vi "Subvi Notify User.vi"(1 "Imaging":bool, 2 "PresentCutsIn":u32, 3 "TotalCutsIn":u32, 4 "NotifyAbout":T1(ring)) -> (0 "Error":bool)   [LabVIEW 2012]
uses:
  ProSCI Global.vi
  <vilib>/Utility/SMTP/NI_SMTPEmail.lvlib
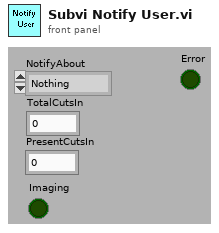
[diagram p1: front panel]
types:
  T1 = enum16{"Nothing", "In Progress", "Aborted", "Completed", "Sec TO"}
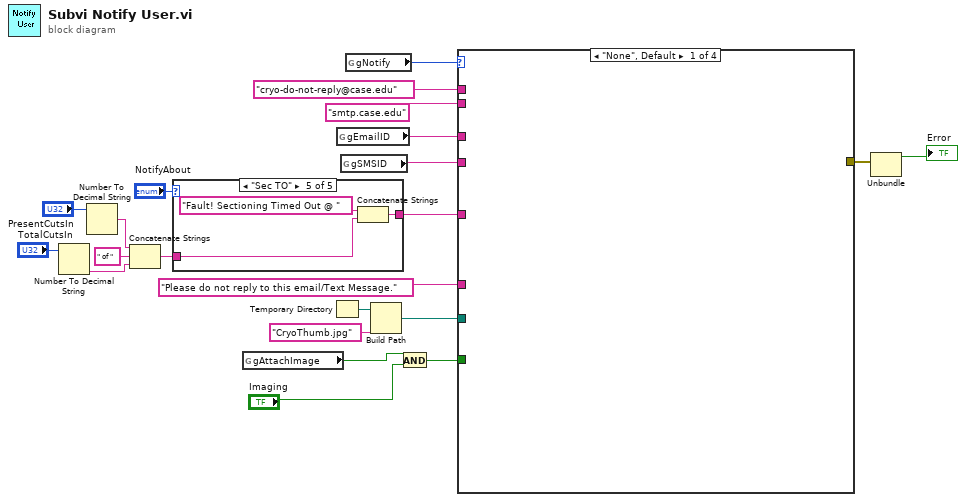
[diagram p0: block diagram]
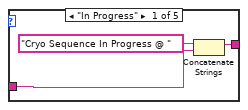
[diagram p2: hidden frame]
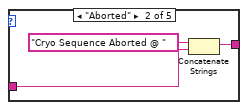
[diagram p3: hidden frame]
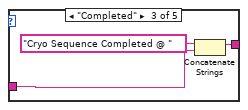
[diagram p4: hidden frame]
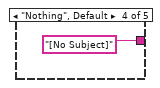
[diagram p5: hidden frame]
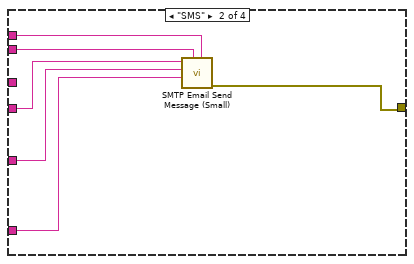
[diagram p6: hidden frame]
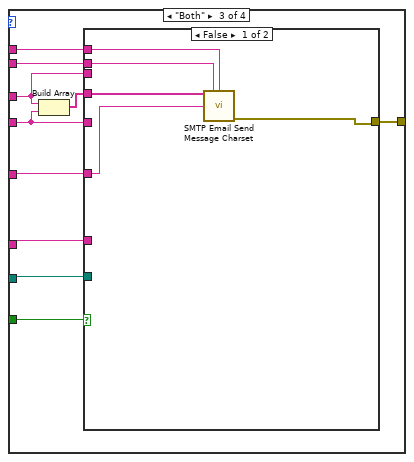
[diagram p7: hidden frame]
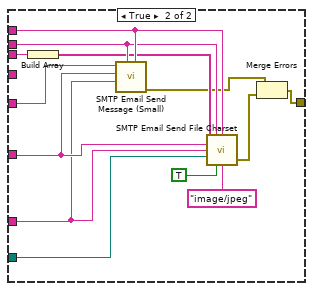
[diagram p8: hidden frame]
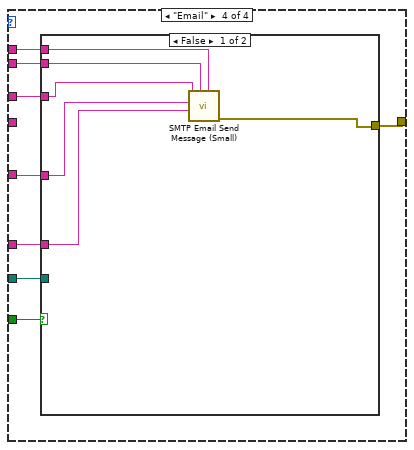
[diagram p9: hidden frame]
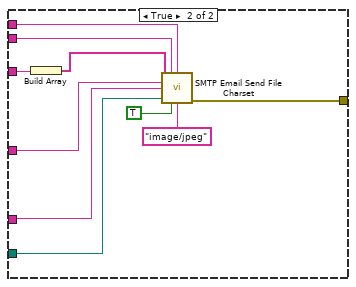
[diagram p10: hidden frame]
diagram:
  n1 = Number To Decimal String(number="TotalCutsIn") -> (decimal integer string=w17:string)  [unwired: 1 out]
  n2 = Number To Decimal String(number="PresentCutsIn") -> (decimal integer string=w19:string)  [unwired: 1 out]
  n3 = Concatenate Strings(w19, " of " ("string"), w17) -> (w16:string)
  n4 = case shown="\"Sec TO\"" "NotifyAbout" {
    tunnel: w16 -> [w24 w27 w30 _ w34]
    tunnel: [w23 w26 w29 "[No Subject]" w33] -> w9
    frame "In Progress" {
      n5 = Concatenate Strings("Cryo Sequence In Progress @ ", w24) -> (w23:string)
    }
    frame "Aborted" {
      n6 = Concatenate Strings("Cryo Sequence Aborted @ ", w27) -> (w26:string)
    }
    frame "Completed" {
      n7 = Concatenate Strings("Cryo Sequence Completed @ ", w30) -> (w29:string)
    }
    frame "Nothing", Default {
    }
    frame "Sec TO" {
      n8 = Concatenate Strings("Fault! Sectioning Timed Out @ " ("Image Name"), w34) -> (w33:string)
    }
  }
  n9 = global read "ProSCI Global.vi" "gAttachImage"() -> (w2:bool)
  n10 = Temporary Directory() -> (w14:path)
  n11 = global read "ProSCI Global.vi" "gEmailID"() -> (w7:string)
  n12 = global read "ProSCI Global.vi" "gSMSID"() -> (w10:string)
  n13 = global read "ProSCI Global.vi" "gNotify"() -> (w15:enum16{"None", "Email", "SMS", "Both"})
  n14 = Build Path(base path=w14, name or relative path="CryoThumb.jpg" ("Image Name")) -> (appended path=w6:path)
  n15 = And(x=w2, y="Imaging") -> (x .and. y?=w3:bool)
  n16 = case shown="\"None\", Default" w15 {
    tunnel: "cryo-do-not-reply@case.edu" -> [_ w41 w50 w76]
    tunnel: "smtp.case.edu" -> [_ w40 w49 w75]
    tunnel: w10 -> [_ w39 w46 _]
    tunnel: w9 -> [_ w38 w47 w73]
    tunnel: "Please do not reply to this email/Text Message." -> [_ w37 w45 w72]
    tunnel: w3 -> [_ _ w51 w77]
    tunnel: w7 -> [_ _ w44 w74]
    tunnel: w6 -> [_ _ w43 w71]
    tunnel: [_ w36 w42 w70] -> w5
    frame "None", Default {
    }
    frame "SMS" {
      n17 = call <vilib>:"SMTP Email Send Message (Small).vi"("return address"=w41, "mail server"=w40, "message"=w37, "subject ([No Subject])"=w38, "recipient"=w39) -> ("error out"=w36:errorcluster)  [unwired: 1 in, 5 out]
    }
    frame "Both" {
      n18 = Build Array(w44, w46) -> (w48:string[])
      n19 = case shown="False" w51 {
        tunnel: w50 -> [w56 w66]
        tunnel: w49 -> [w55 w65]
        tunnel: w48 -> [w54 _]
        tunnel: w47 -> [w53 w62]
        tunnel: w46 -> [_ w69]
        tunnel: w45 -> [_ w61]
        tunnel: w44 -> [_ w64]
        tunnel: w43 -> [_ w60]
        tunnel: [w52 w57] -> w42
        frame False {
          n20 = call <vilib>:"SMTP Email Send Message Charset.vi"("recipients"=w54, "mail server"=w55, "return address"=w56, "message"=w53) -> ("error out"=w52:errorcluster)  [unwired: 3 in, 8 out]
        }
        frame True {
          n21 = Build Array(w64) -> (w63:string[])
          n22 = call <vilib>:"SMTP Email Send Message (Small).vi"("return address"=w66, "mail server"=w65, "message"=w61, "subject ([No Subject])"=w62, "recipient"=w69) -> ("error out"=w59:errorcluster)  [unwired: 1 in, 5 out]
          n23 = call <vilib>:"SMTP Email Send File Charset.vi"("recipients"=w63, "mail server"=w65, "return address"=w66, "subject ([No Subject])"=w62, "message"=w61, "file path"=w60, "binary? (F)"=TRUE, "MIME content-type (application/octet-stream)"="image/jpeg") -> ("error out"=w58:errorcluster)  [unwired: 2 in, 5 out]
          n24 = Merge Errors(w59, w58) -> (w57:errorcluster)
        }
      }
    }
    frame "Email" {
      n25 = case shown="False" w77 {
        tunnel: w76 -> [w83 w93]
        tunnel: w75 -> [w82 w92]
        tunnel: w74 -> [w81 w91]
        tunnel: w73 -> [w80 w89]
        tunnel: w72 -> [w79 w88]
        tunnel: w71 -> [_ w87]
        tunnel: [w78 w84] -> w70
        frame False {
          n26 = call <vilib>:"SMTP Email Send Message (Small).vi"("return address"=w83, "mail server"=w82, "message"=w79, "subject ([No Subject])"=w80, "recipient"=w81) -> ("error out"=w78:errorcluster)  [unwired: 1 in, 5 out]
        }
        frame True {
          n27 = Build Array(w91) -> (w90:string[])
          n28 = call <vilib>:"SMTP Email Send File Charset.vi"("recipients"=w90, "mail server"=w92, "return address"=w93, "subject ([No Subject])"=w89, "message"=w88, "file path"=w87, "binary? (F)"=TRUE, "MIME content-type (application/octet-stream)"="image/jpeg") -> ("error out"=w84:errorcluster)  [unwired: 2 in, 5 out]
        }
      }
    }
  }
  n29 = Unbundle(w5) -> ("status"=→"Error":bool)  [unwired: 2 out]
